vi "Rx Inline Wait.vi"(8 "error in (no error)":errorcluster, 11 "Framework in":refnum<class "Framework.lvclass">) -> (0 "error out":errorcluster, 3 "Framework out":refnum<class "Framework.lvclass">)   [LabVIEW 2017, in "DSF Core.lvlib" / "Framework.lvclass"]
uses:
  Framework.lvclass
  Framework.lvclass/Framework.ctl
  Plugin/Plugin.lvclass/Plugin.ctl
  Transfer Group/Transfer Group.lvclass/Transfer Group.ctl
  Timing/Timing.lvclass/Timing.ctl
  <vilib>/NI/Memory Manager/Classes/Pointer/Pointer.lvclass/Pointer.ctl
  Transfer Group/Wait For Previous.vi
  Transfer Group/Update Status.vi
  Transfer Group/Retrieve from FIFO.vi
  Transfer Group/Get Iteration.vi
  Transfer Group Status/Write Status.vi
  Transfer Group/Read Return FIFO.vi
  Transfer Group/Increment Late Count.vi
  Timing/Get Iteration.vi
  Transfer Group Status/Write Status.vi/dcfa478e-d62b-496d-bee8-da79212ebf54.vi
  Transfer Group Status/Write Status.vi/dcfa478e-d62b-496d-bee8-da79212ebf54.vi/2395fb35-3986-41f2-8d0d-0c3dcc4c836d.vi
  <vilib>/NI/Memory Manager/Classes/Pointer/Get Address.vi
  <vilib>/NI/Memory Manager/Classes/Pointer/Check Size (0D).vi
  <vilib>/NI/Memory Manager/Classes/Pointer/Errors.vi
  <vilib>/NI/Memory Manager/Classes/Pointer/Out of Bounds.vi
  <vilib>/NI/Memory Manager/Classes/Pointer/Get Size.vi
  <vilib>/NI/Memory Manager/VIs/Source.Write.String.vi
  <vilib>/NI/Memory Manager/Classes/Pointer/Write Pointer Size.vi
  <vilib>/NI/Memory Manager/Classes/Pointer/Create Error.vi
  <vilib>/NI/Memory Manager/VIs/Source.Write.Scalar.Base10.vi
  <vilib>/NI/Memory Manager/VIs/Source.Write.Scalar.Base10 (U64).vi
  <vilib>/NI/Memory Manager/VIs/New Error Cluster Constant.vi
  <vilib>/NI/Memory Manager/VIs/New Error Cluster Constant (512B).vi
  <vilib>/NI/Memory Manager/VIs/Error Cluster.Set Status.vi
  <vilib>/NI/Memory Manager/VIs/Error Cluster.Set Code.vi
  <vilib>/NI/Memory Manager/VIs/Error Cluster.Set VI Source.vi
  <vilib>/NI/Memory Manager/Constants/Constants.vi
  <vilib>/NI/Memory Manager/Constants/Library Name.vi
  <vilib>/NI/Memory Manager/Classes/Pointer/Pointer Error Info.vi
  <vilib>/NI/Memory Manager/Constants/Pointer Class Name.vi
  Transfer Group Status/Transfer Group Status.lvclass
  C:/Program Files (x86)/National Instruments/LabVIEW 2017/vi.lib/NI/Memory Manager/Classes/Pointer/Pointer.lvclass
  Transfer Group/Errors.vi
  Transfer Group/Return Timeout Error.vi
  Transfer Group/Invalid Iteration Error.vi
  Plugin/Plugin.lvclass
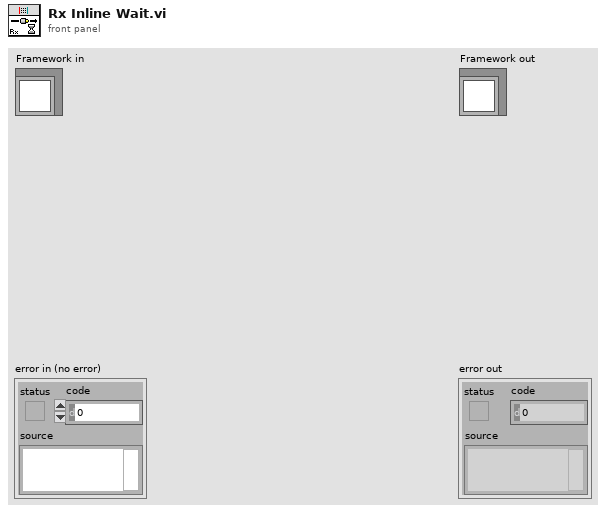
[diagram p1: front panel]
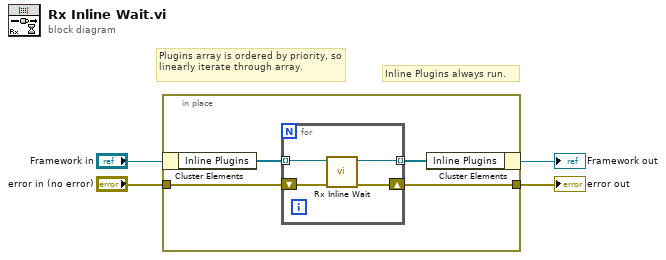
[diagram p0: block diagram]
diagram:
  # "Inline Plugins always run."
  # "Plugins array is ordered by priority, so linearly iterate through array."
  n1 = in-place {
    in-place-border: "error in (no error)" -> [w8]
    in-place-border: [w7] -> w3
    n2 = in-place-cluster #1("Framework in") -> ("Inline Plugins"=w6:refnum<class "Plugin.lvclass">[])
    n3 = for {
      tunnel: w6 -> [w9] mode=indexing
      tunnel: [w12] -> w5 mode=indexing
      shift-right: [w11] -> w7
      shift-left: w8 -> [w10]
      n4 = call "Rx Inline Wait.vi"("error in (no error)"=w10, "Plugin in"=w9) -> ("error out"=w11:errorcluster, "Plugin out"=w12:refnum<class "Plugin.lvclass">)  [unwired: 8 in]
    }
    n5 = in-place-cluster #1("Inline Plugins"=w5) -> (→"Framework out":refnum<class "Framework.lvclass">)
  }
  "error out" <- w3
